vi "U3 DAC Output from File.vi"() -> ()   [LabVIEW 2021]
uses:
  <vilib>/Utility/file.llb/Read From Spreadsheet File (DBL).vi
panel:
  out "Array Size":i32
  out "Iteration":i32
  out "Udate Array from File":sgl[](array[numeric])
  in  "Update Interval (ms)":u32=1000
  out "Error":string
  out "Waveform Chart":dbl(graph)
  in  "Stop":bool
  # "Updates DAC0 at the specified update interval in order to build time series waveforms.  The\nupdate interval is set to 1000 ms by default, but can be set lower based on the execution times\ndiscussed in Section 3.1 of the U3 User's Guide.  Uses the first found U3.\n\nWith a software timed application such as this, you might be able to reduce timing jitter (caused\nby the operating system) by increasing the priority of this process (labview.exe) in Windows\nTask Manager."
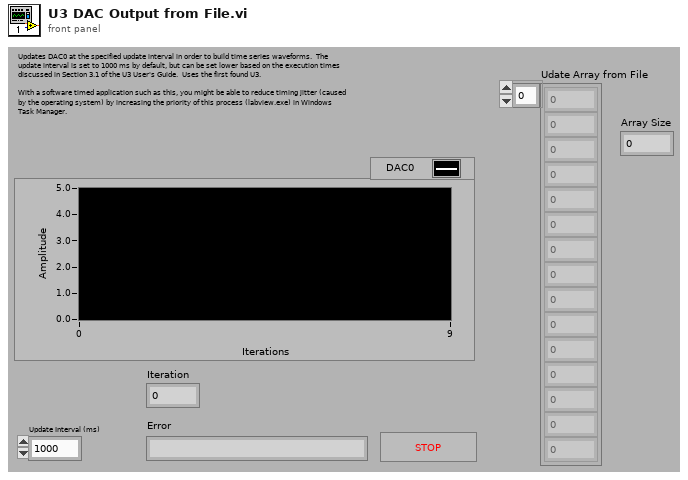
[diagram p1: front panel]
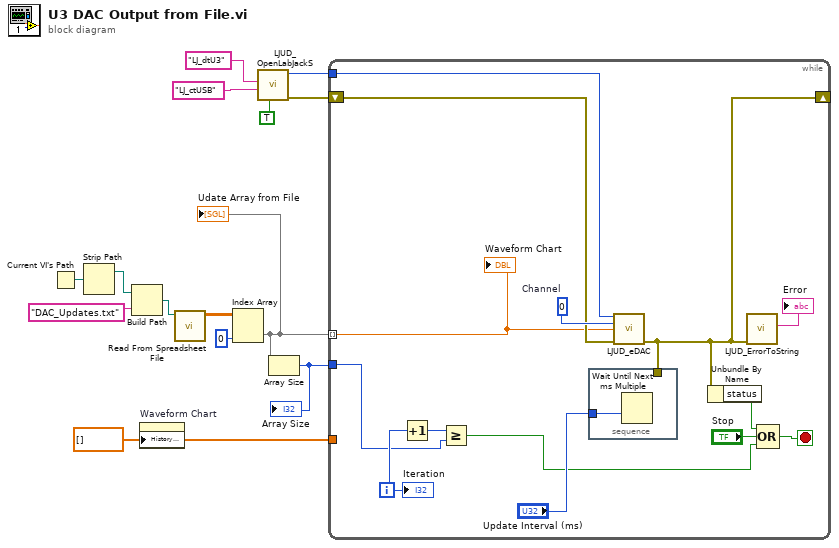
[diagram p0: block diagram]
diagram:
  w1 = sgl[] [] ("History Data")
  n1 = Current VI's Path() -> (path=w3:path)
  n2 = Strip Path(path=w3) -> (stripped path=w2:path)  [unwired: 1 out]
  n3 = Build Path(base path=w2, name or relative path="DAC_Updates.txt" ("file path (dialog if empty)")) -> (appended path=w4:path)
  n4 = property on="Waveform Chart" class="WFChart (strict)"("History Data"=w1) -> ()  [unwired: 2 in, 2 out]
  n5 = call-poly <vilib>:"Read From Spreadsheet File.vi"("file path (dialog if empty)"=w4) -> ("all rows"=w9:dbl[][])  [unwired: 6 in, 4 out]
  n6 = Index Array(array=w9, index (col)=0 ("disabled index (col)")) -> (element=w7:dbl[])  [unwired: 1 in]
  "Udate Array from File" <- w7
  n7 = call "LJUD_OpenLabJackS.vi"("FirstFound"=TRUE, "ConnectionType"="LJ_ctUSB", "DeviceType"="LJ_dtU3") -> ("error out"=w11:errorcluster, "Handle"=w10:i32)  [unwired: 6 in, 1 out]
  n8 = Array Size(array=w7) -> (size(s)=w6:i32)
  "Array Size" <- w6
  n9 = while {
    tunnel: w10 -> [w21]
    shift-left: w11 -> [w23]
    shift-right: [w22] -> _
    tunnel: w7 -> [w19] mode=indexing
    tunnel: w6 -> [w16]
    tunnel: w1 -> [_]
    i -> [w17]
    stop <- w25 stop-if-true
    w24 = 0  # Channel
    n10 = Increment(x=w17) -> (x+1=w18:i32)
    n11 = Greater Or Equal?(x=w18, y=w16) -> (x >= y?=w15:bool)
    n12 = call "LJUD_eDAC.vi"("Handle In"=w21, "Channel"=w24, "Voltage"=w19, "error in"=w23) -> ("error out"=w22:errorcluster)  [unwired: 10 in, 1 out]
    n13 = stacked-sequence {
      tunnel: "Update Interval (ms)" -> [w29]
      tunnel: w22 -> [_]
      frame #0 {
        n14 = Wait Until Next ms Multiple(millisecond multiple=w29) -> ()  [unwired: 1 out]
      }
    }
    n15 = Unbundle By Name(w22) -> ("status"=w26:bool)
    n16 = call "LJUD_ErrorToString.vi"("error in"=w22) -> ("String"=→"Error":string)  [unwired: 10 in]
    n17 = Compound Arithmetic op=OR(w26, "Stop", w15) -> (w25:bool)
    "Waveform Chart" <- w19
    "Iteration" <- w17
  }
